vi "ContinueScan.vi"(8 "error in":errorcluster, 10 "input cluster":T1={"Scanning Segments Left"=0, "Scanning"=FALSE, "Path"=path "", "FileName"="", "Scan Segments"=0, "Step Time (us)"=100, "Polarity"=enum."Positive", "Direction"=enum."Forward", "Steps"=1, "Image"=[]} {"Steps" min=1 max=10000 step=1 scale=1.0..10000.0; "Step Time (us)" min=100 step=10 scale=100.0..10000.0; "Scan Segments" max=100 step=1 scale=0.0..100.0}, 11 "Message Enqueuer in":refnum<class "Message Enqueuer.lvclass">) -> (0 "error out":errorcluster, 2 "output cluster":T1={"Scanning Segments Left"=0, "Scanning"=FALSE, "Path"=path "", "FileName"="", "Scan Segments"=0, "Step Time (us)"=100, "Polarity"=enum."Positive", "Direction"=enum."Forward", "Steps"=1, "Image"=[]} {"Steps" min=1 max=10000 step=1 scale=1.0..10000.0; "Step Time (us)" min=100 step=10 scale=100.0..10000.0; "Scan Segments" max=100 step=1 scale=0.0..100.0})   [LabVIEW 2023, in "InterferometryUI.lvlib" / "InterferometryUI.lvclass"]
uses:
  InterferometryUI.lvclass
  <vilib>/ActorFramework/Message Enqueuer/Message Enqueuer.lvclass
  InterferometryUIPublicData.ctl
  ArduinoTranslationStageUI/ArduinoTranslationStageActor/ArduinoTranslationStage Messages/MoveBySteps Msg/MoveBySteps Msg.lvclass/MoveBySteps Msg.ctl
  <vilib>/ActorFramework/Message Enqueuer/Message Enqueuer.lvclass/Message Enqueuer.ctl
  <vilib>/ActorFramework/Message Enqueuer/Enqueue.vi
  ArduinoTranslationStageUI/ArduinoTranslationStageActor/ArduinoTranslationStage Messages/MoveBySteps Msg/MoveBySteps Msg.lvclass
  Applications/National Instruments/LabVIEW 2023 64-bit/vi.lib/ActorFramework/Message/Message.lvclass
  <vilib>/ActorFramework/Message Priority Queue/Priority Enqueue.vi
  InterferometryUI.lvclass/InterferometryUI.ctl
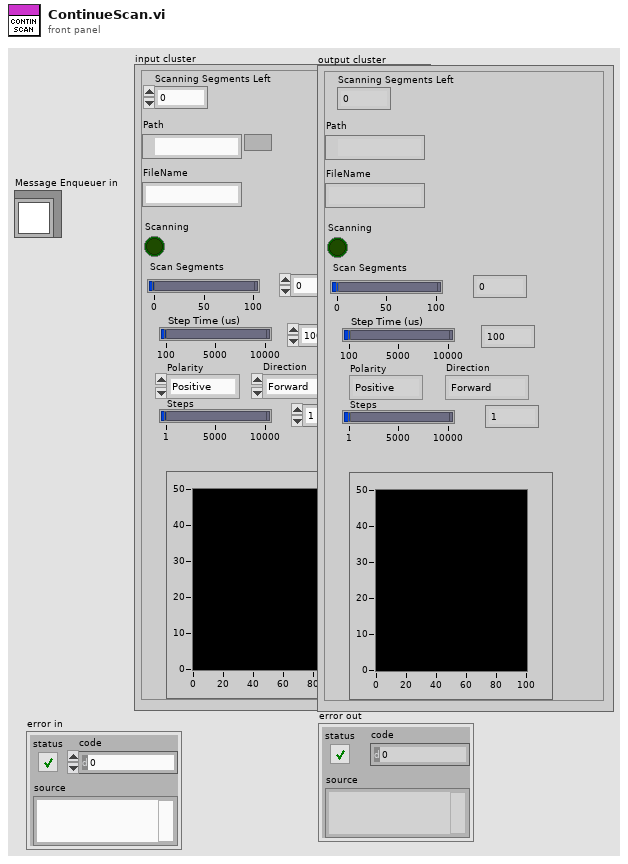
[diagram p1: front panel]
types:
  T1 = typedef "InterferometryUIPublicData.ctl" = cluster{"Scanning Segments Left":u16, "Scanning":bool, "Path":path, "FileName":string, "Scan Segments":u32, "Step Time (us)":u32, "Polarity":enum16{"Positive", "Negative"}, "Direction":enum16{"Forward", "Backwards"}, "Steps":u32, "Image":u16[][]}
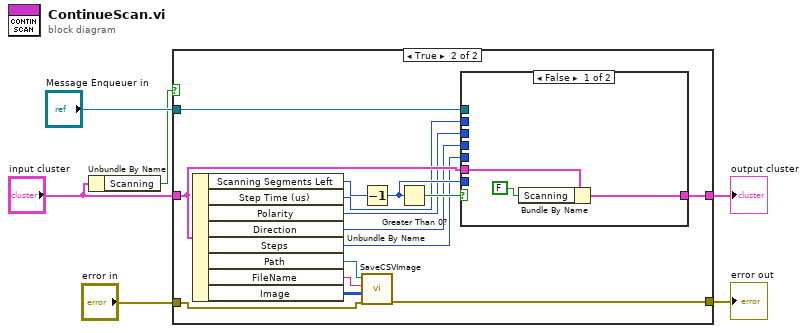
[diagram p0: block diagram]
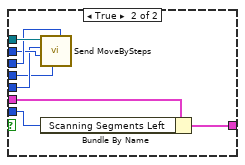
[diagram p3: hidden frame]
diagram:
  n1 = Unbundle By Name("input cluster") -> ("Scanning"=w5:bool)
  n2 = case shown="True" w5 {
    tunnel: [w8 w23] -> w3
    tunnel: "Message Enqueuer in" -> [_ w20]
    tunnel: "input cluster" -> [w8 w18]
    tunnel: [w7 w10] -> w2
    tunnel: "error in" -> [w7 w9]
    frame False {
    }
    frame True {
      n3 = Unbundle By Name(w18) -> ("Scanning Segments Left"=w19:u16, "Step Time (us)"=w16:u32, "Polarity"=w17:enum16{"Positive", "Negative"}, "Direction"=w14:enum16{"Forward", "Backwards"}, "Steps"=w15:u32, "Path"=w13:path, "FileName"=w12:string, "Image"=w11:u16[][])
      n4 = Decrement(x=w19) -> (x-1=w22:u16)
      n5 = call "SaveCSVImage.vi"("error in (no error)"=w9, "Image"=w11, "FileName"=w12, "Path"=w13) -> ("error out"=w10:errorcluster)  [unwired: 7 in]
      n6 = Greater Than 0?(x=w22) -> (x > 0?=w21:bool)
      n7 = case shown="False" w21 {
        tunnel: [w25 w28] -> w23
        tunnel: w22 -> [_ w34]
        tunnel: w20 -> [_ w33]
        tunnel: w18 -> [w24 w27]
        tunnel: w17 -> [_ w32]
        tunnel: w16 -> [_ w31]
        tunnel: w15 -> [_ w30]
        tunnel: w14 -> [_ w29]
        frame False {
          n8 = Bundle By Name(cluster=w24, "Scanning"=FALSE) -> (w25:T1)
        }
        frame True {
          n9 = call "Send MoveBySteps.vi"("Polarity"=w32, "Direction"=w29, "Speed"=w31, "Steps"=w30, "Message Enqueuer"=w33) -> ()  [unwired: 5 in, 2 out]
          n10 = Bundle By Name(cluster=w27, "Scanning Segments Left"=w34) -> (w28:T1)
        }
      }
    }
  }
  "output cluster" <- w3
  "error out" <- w2
